vi "Set Report Margins.vi"(0 "report in":refnum<class "NI_HTML.lvclass">, 5 "margins (1.00)":T1={"top"=1.0, "left"=1.0, "right"=1.0, "bottom"=1.0} {"right" format="%.2f"; "bottom" format="%.2f"; "top" format="%.2f"; "left" format="%.2f"}, 9 "measurement system (default)":u16(ring) items=["Default", "US", "Metric"], 11 "error in (no error)":errorcluster) -> (4 "report out":refnum<class "NI_HTML.lvclass">, 10 "page width (Word)":sgl format="%.2f", 15 "error out":errorcluster)   [LabVIEW 2020, in "NI_HTML.lvclass"]
doc: "Sets the margins of the specified report."
uses:
  <vilib>/Utility/NIReport.llb/HTML/NI_HTML.lvclass
  <vilib>/Utility/NIReport.llb/HTML/NI_HTML.lvclass/NI_HTML.ctl
  <vilib>/Utility/NIReport.llb/NI_ReportGenerationCore.lvlib
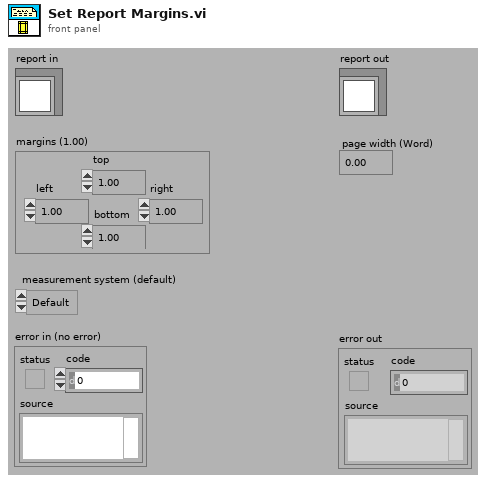
[diagram p1: front panel]
types:
  T1 = cluster{"top":dbl, "left":dbl, "right":dbl, "bottom":dbl}
  T2 = typedef "NI_ReportGenerationCore.lvlib/HTML Report Data.ctl" = cluster{"Body Text":string, "Font Tag":string, "Title Text":string, "Header Text":string, "Footer Text":string, "Image List":path[]}
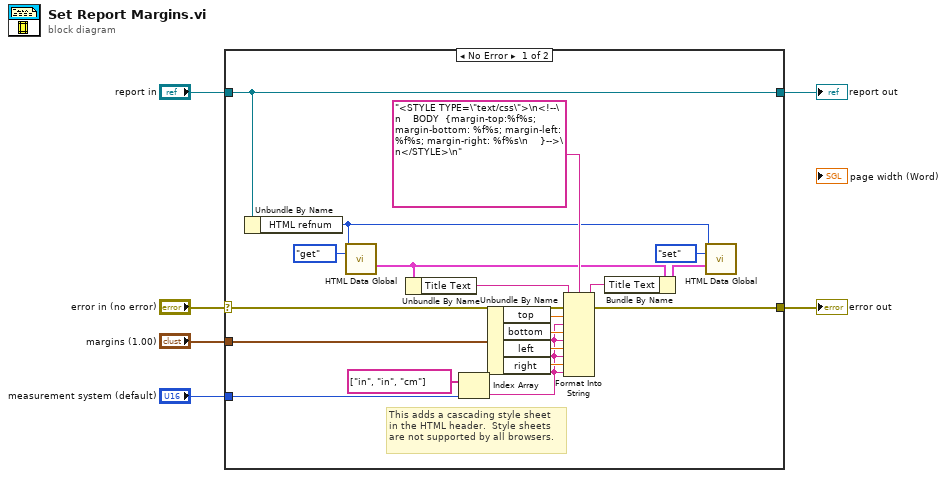
[diagram p0: block diagram]
diagram:
  n1 = case shown="No Error" "error in (no error)" {
    selector: "error in (no error)" -> [w14 w27]
    tunnel: [w13 w27] -> w5
    tunnel: [w11 w26] -> w3
    tunnel: "report in" -> [w11 w26]
    tunnel: "margins (1.00)" -> [w16 _]
    tunnel: "measurement system (default)" -> [w15 _]
    frame No Error {
      # "This adds a cascading style sheet\nin the HTML header.  Style sheets\nare not supported by all browsers."
      n2 = Unbundle By Name(w11) -> ("HTML refnum"=w7:u32)
      n3 = call <vilib>:"HTML Data Global.vi"("HTML refnum"=w7, "menu"=enum16{"init", "get", "set", "delete"}."get") -> ("HTML report data out"=w9:T2)  [unwired: 1 in, 12 out]
      n4 = Unbundle By Name(w9) -> ("Title Text"=w21:string)
      n5 = Index Array(array=string[] ["in", "in", "cm"] ("Array Constant"), index=w15) -> (element=w18:string)
      n6 = Unbundle By Name(w16) -> ("top"=w22:dbl, "bottom"=w23:dbl, "left"=w24:dbl, "right"=w25:dbl)
      n7 = Format Into String(format string="<STYLE TYPE=\"text/css\">\n<!--\n    BODY  {margin-top:%f%s; margin-bottom: %f%s; margin-left: %f%s; margin-right: %f%s\n    }-->\n</STYLE>\n", initial string=w21, error in=w14, w22, w18, w23, w18, w24, w18, w25, w18) -> (resulting string=w20:string, error out=w13:errorcluster)
      n8 = Bundle By Name(cluster=w9, "Title Text"=w20) -> (w8:T2)
      n9 = call <vilib>:"HTML Data Global.vi"("HTML refnum"=w7, "menu"=enum16{"init", "get", "set", "delete"}."set", "HTML report data in"=w8) -> ()  [unwired: 13 out]
    }
    frame Error {
    }
  }
  "error out" <- w5
  "report out" <- w3
